vi "MAIN.vi"() -> ()   [LabVIEW 2020]
uses:
  GLOBALS.vi
panel:
  in  "Period 3":i64=20
  in  "Tab Control":enum32{"Page 1", "Page 2"}(tab)
  in  "reset":bool
  in  "Tecnica":bool
  out "PLOT_ALL":dynamicdata(graph)
  out "chaveamento":dbl
  out "HISTERESE":dbl(graph)
  out "termico":dbl
  out "TERMICO":dbl(graph)
  out "kalman_fused":dbl
  out "KALMAN_FUSED":dbl(graph)
  out "pitot":dbl
  out "Pitot? 2":bool
  out "Térmico?":bool
  out "Pitot?":bool
  out "PITOT":dbl(graph)
  in  "TERMICO Noise Amplitude":dbl=0.8
  in  "PITOT Noise Amplitude":dbl=2.0
  in  "Input":dbl(slide)=8.0 min=0.0 max=100.0 step=0.1 scale=0.0..100.0
  out "error":errorcluster
  in  "M":i32=10 min=2 max=100
  out "Térmico?":bool
  in  "hmin":dbl=8.0 min=5.0 max=20.0 step=1.0
  in  "hmax":dbl=11.0 min=6.0 max=14.0 step=1.0
  in  "stop":bool
  in  "gain delay termico\n[0,100]":dbl=93.0 min=0.0 max=100.0 step=1.0
  in  "Limpar_Graficos":bool
  in  "gain delay pitot [0,100]":dbl=50.0 min=0.0 max=100.0 step=1.0
  in  "PRINT":bool
  out "Kalman?":bool=TRUE
  in  "Ts [ms]":u32=200
  in  "saturacao_termico":dbl=15.0 format="%#_13g"
  # "Medidas Puras"
  # "Medidas Fundidas"
  # "Configurações\nda simulação"
  # "Chaveamento\ncom Histerese"
  # "Filtro de \nKalman"
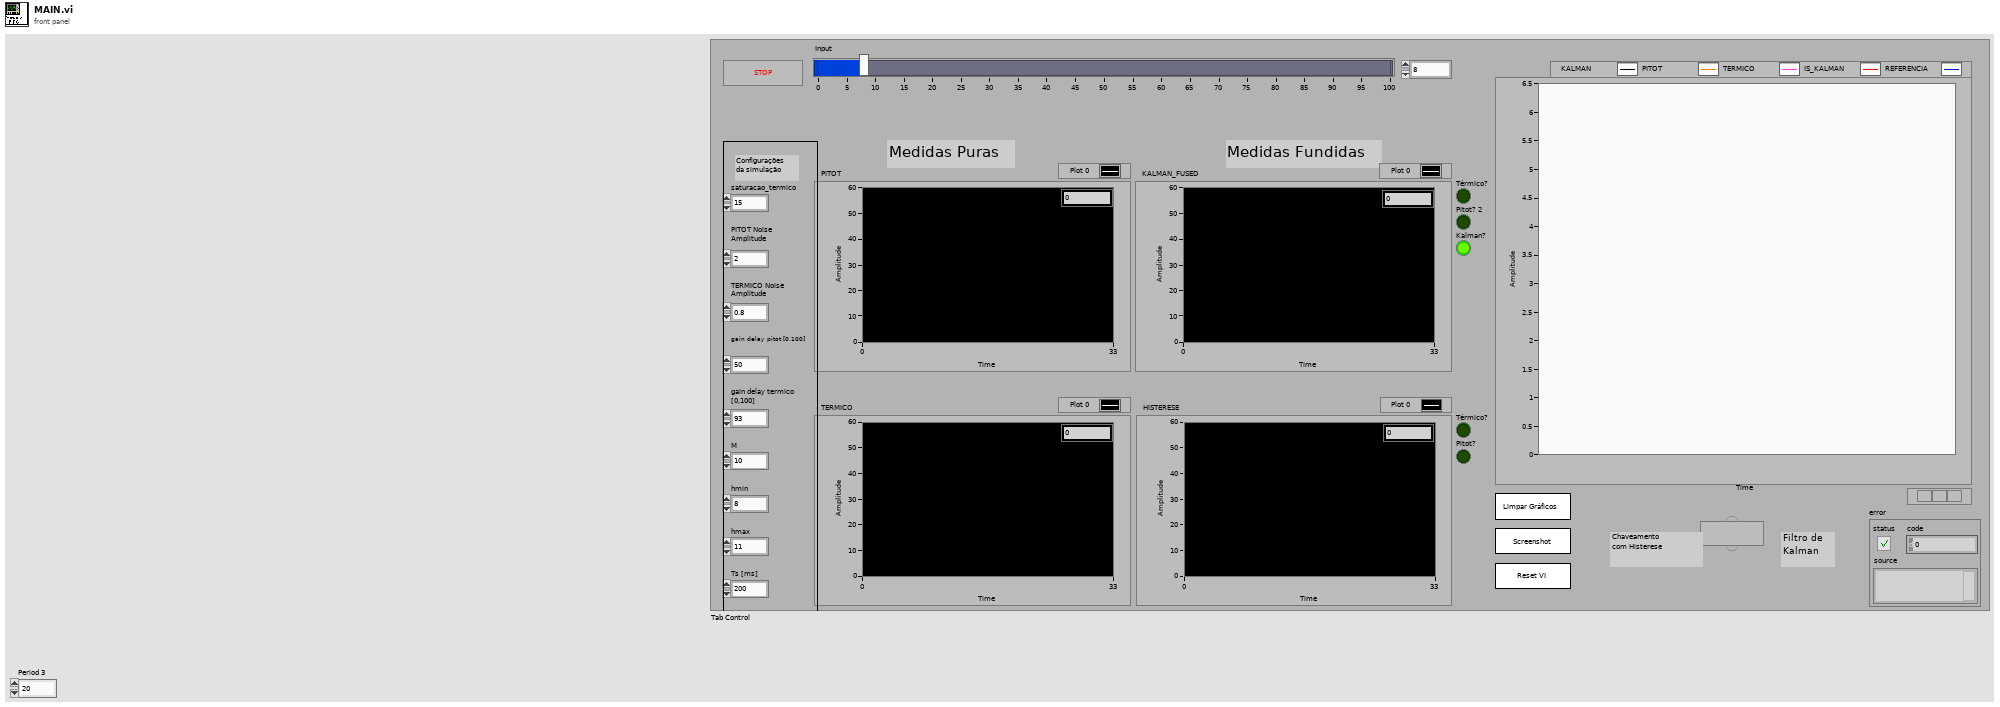
[diagram p1: front panel]
types:
  T1 = typedef "imagedata.ctl" = cluster{"image type":i32, "image depth":i32, "image":u8[], "mask":u8[], "colors":u32[], "Rectangle":cluster{"left":i16, "top":i16, "right":i16, "bottom":i16}}
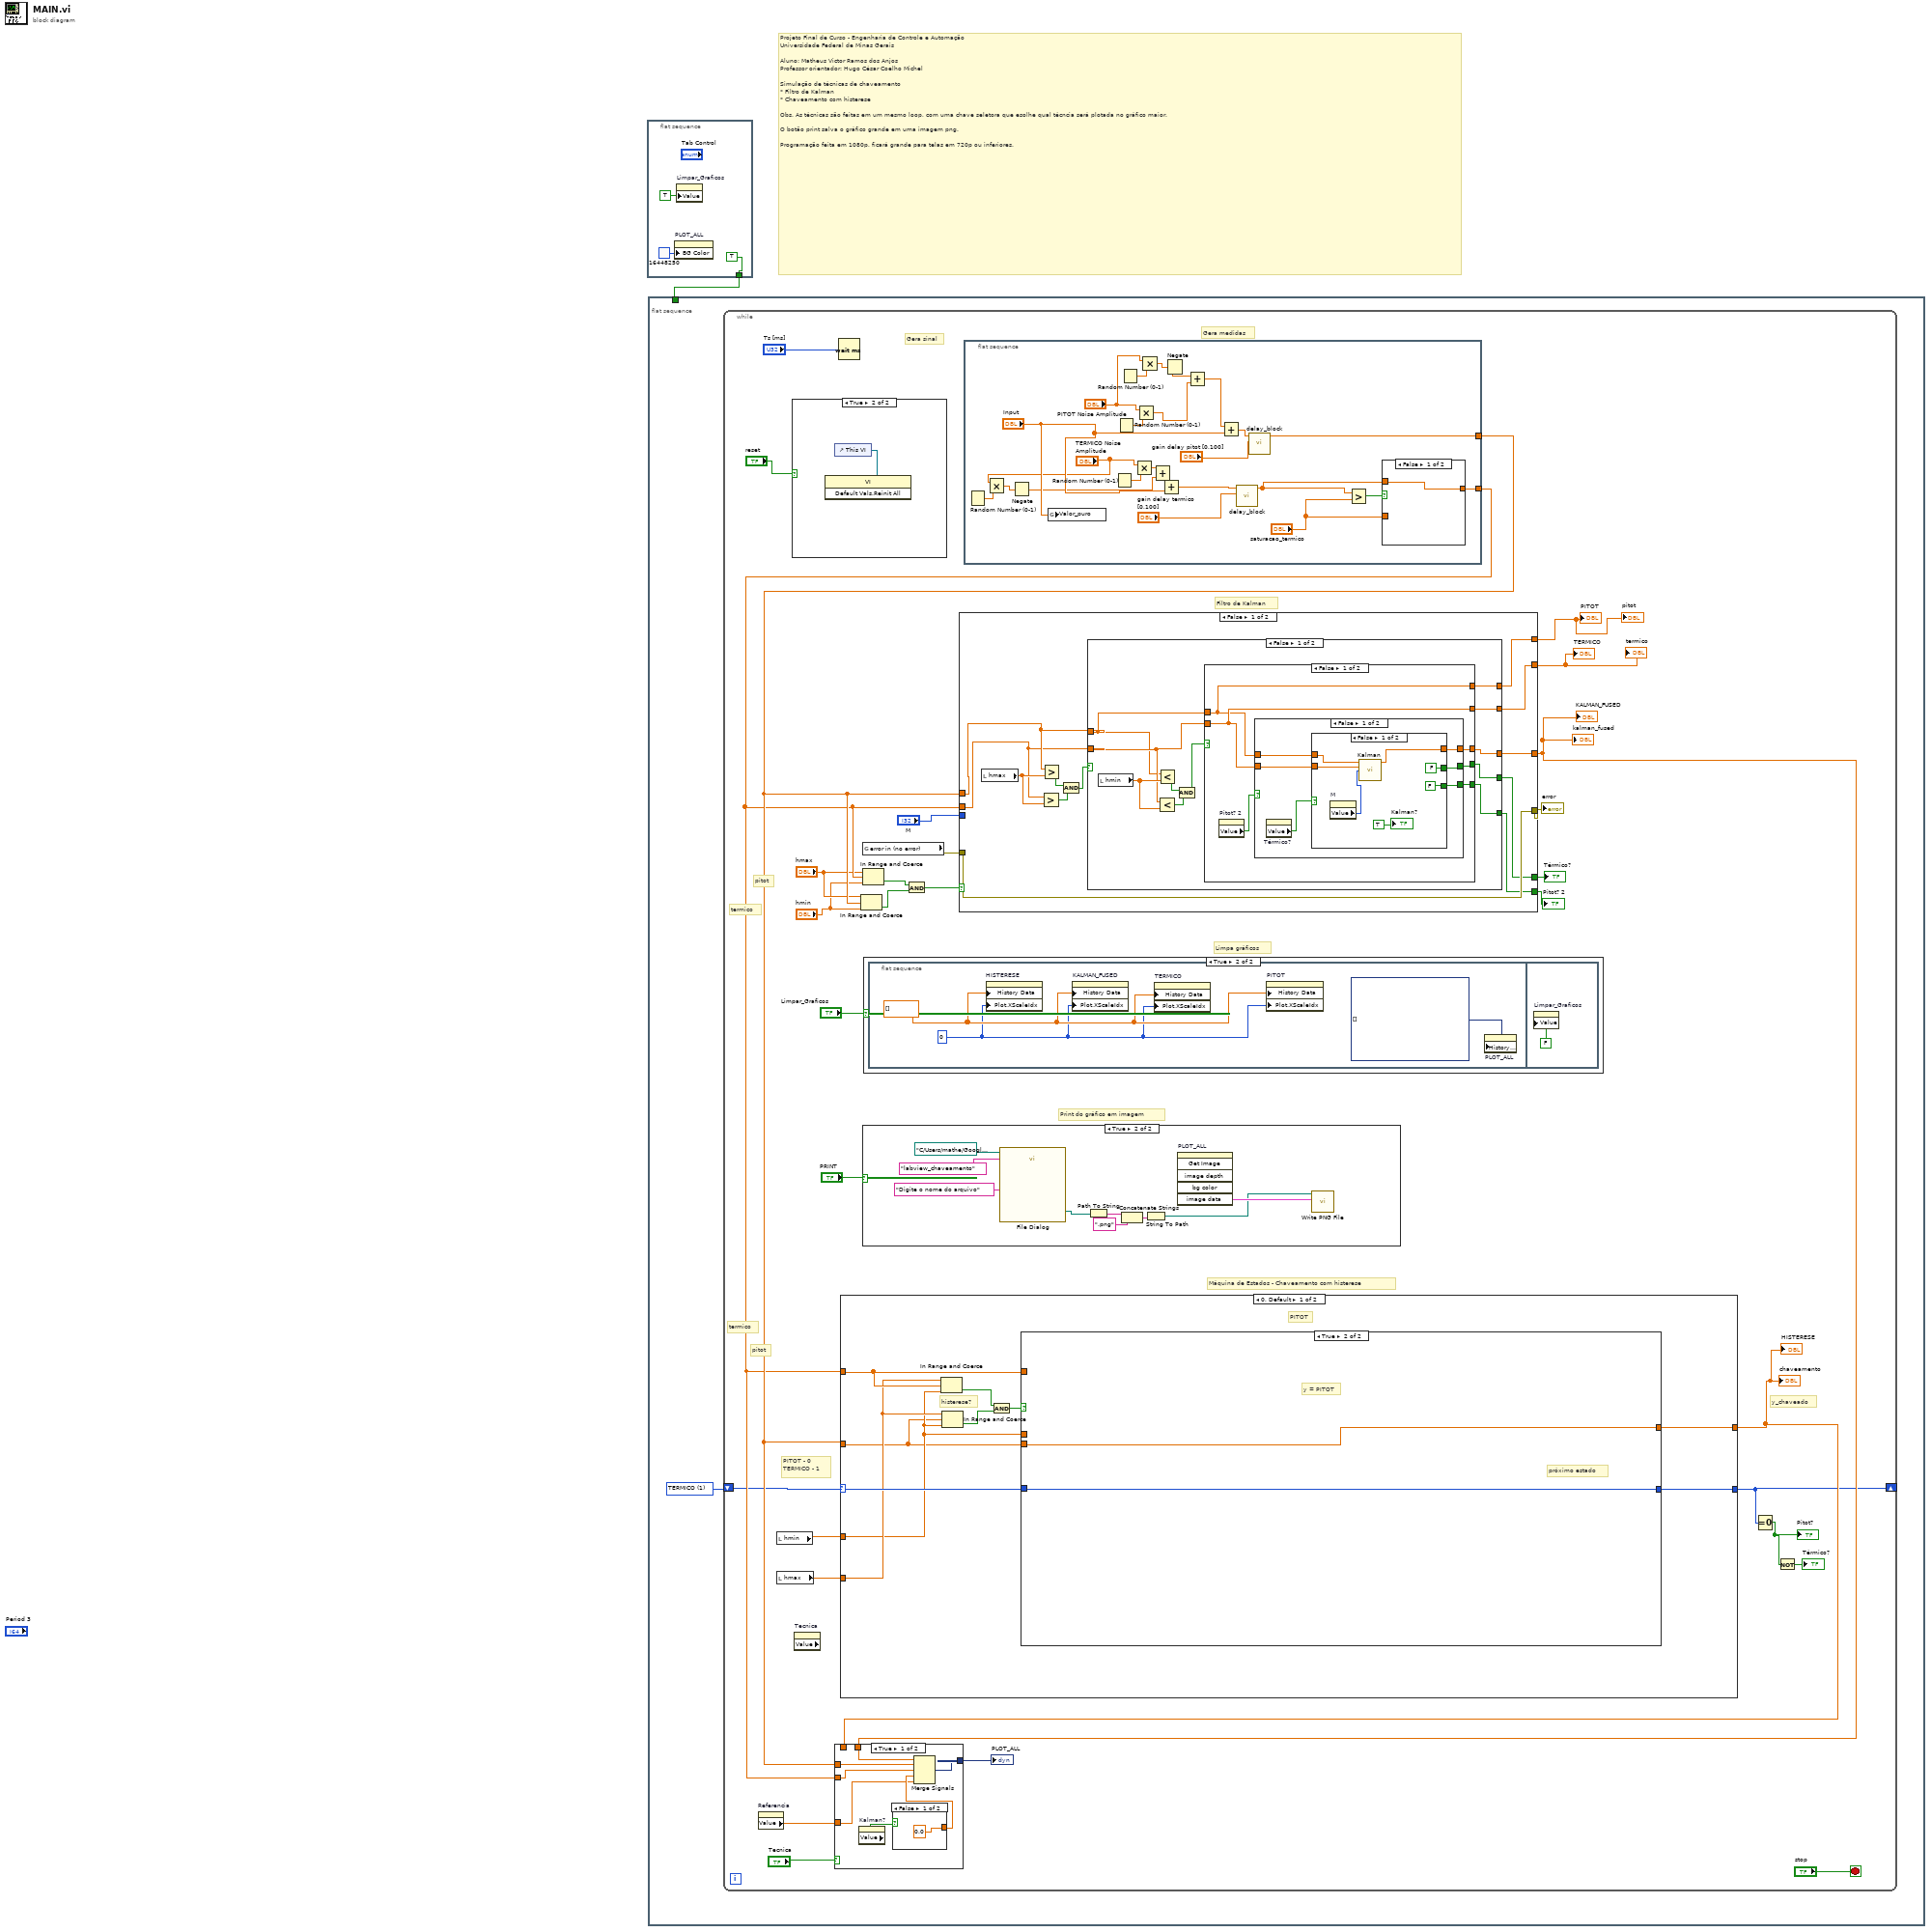
[diagram p0: block diagram]
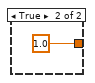
[diagram p4: hidden frame]
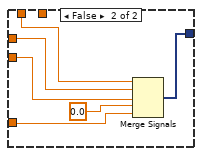
[diagram p5: hidden frame]
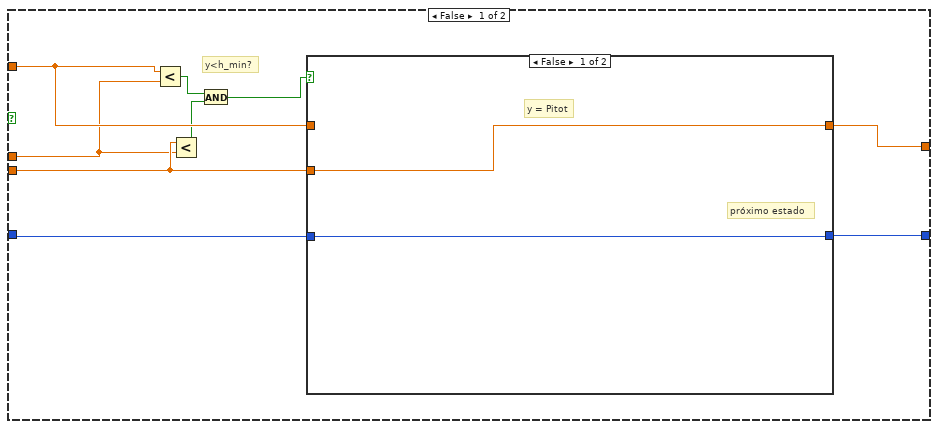
[diagram p6: hidden frame]
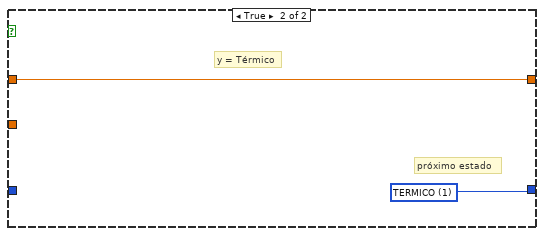
[diagram p7: hidden frame]
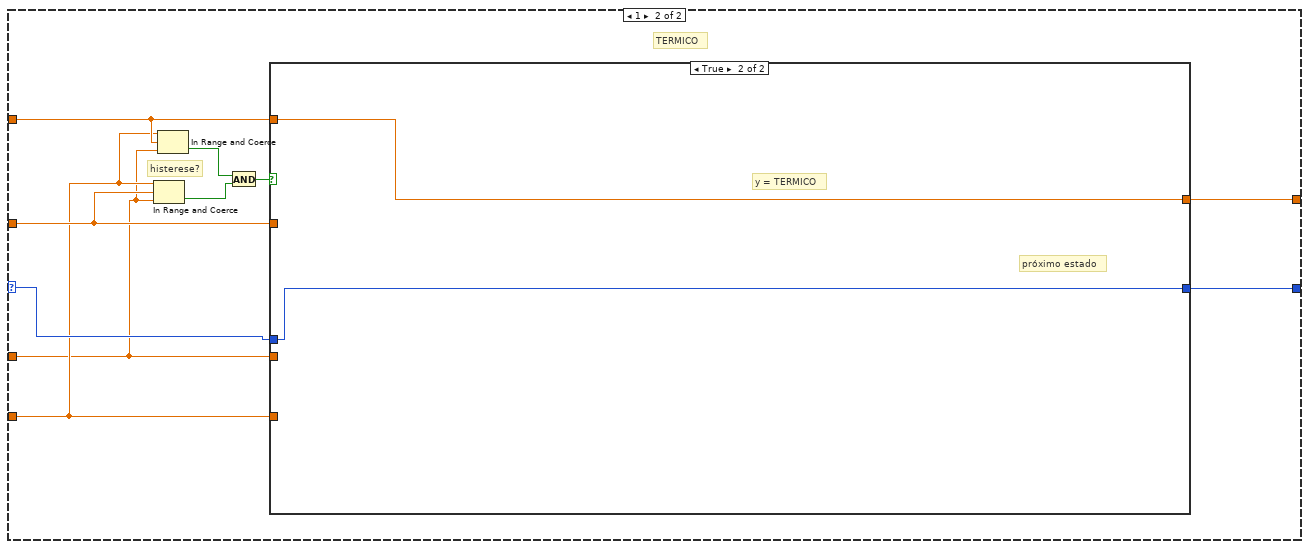
[diagram p8: hidden frame]
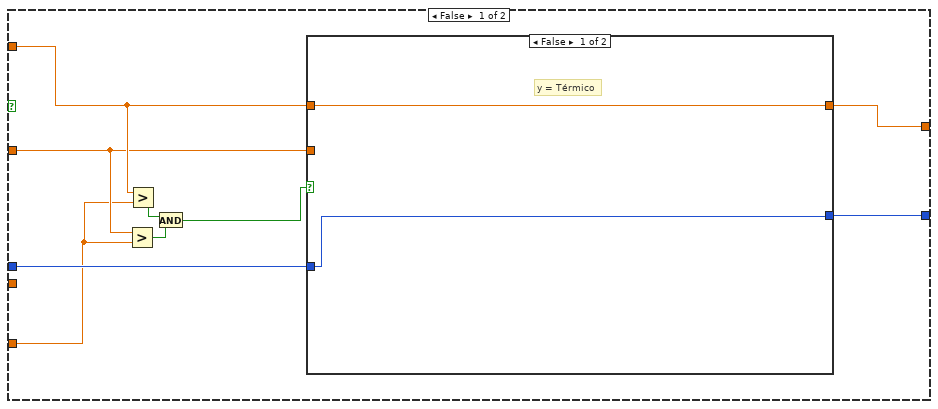
[diagram p9: hidden frame]
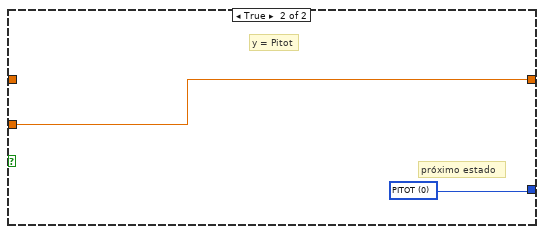
[diagram p10: hidden frame]
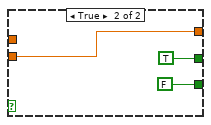
[diagram p13: hidden frame]
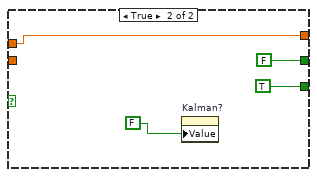
[diagram p14: hidden frame]
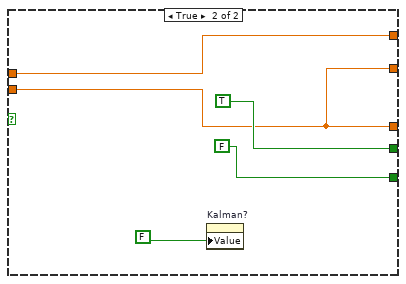
[diagram p15: hidden frame]
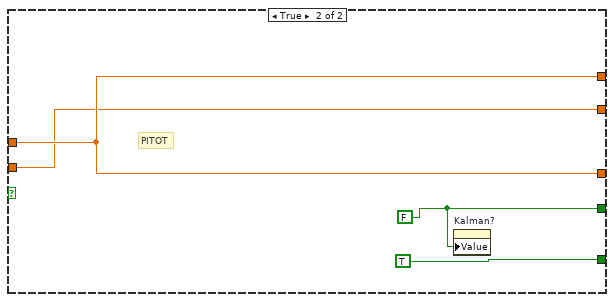
[diagram p16: hidden frame]
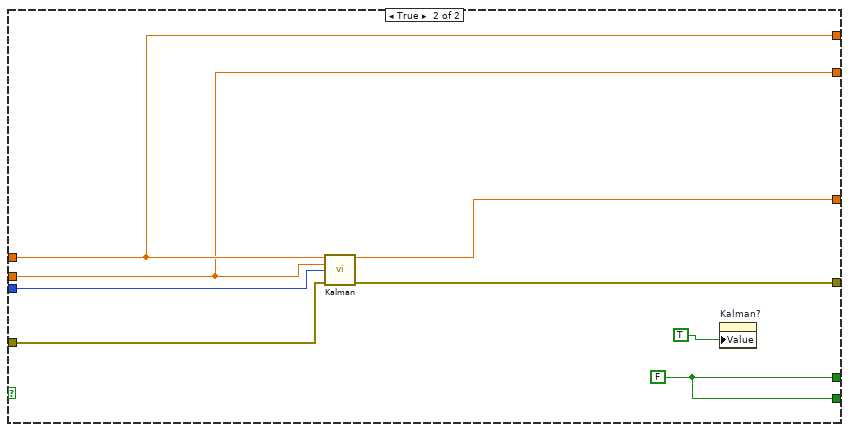
[diagram p17: hidden frame]
diagram:
  # "Projeto Final de Curso - Engenharia de Controle e Automação\nUniversidade Federal de Minas Gerais\n\nAluno: Matheus Victor Ramos dos Anjos\nProfessor orientador: Hugo César Coelho Michel\n\nSimulação de técnicas de chaveamento\n* Filtro de Kalman\n* Chaveamento com histerese\n\nObs. As técnicas são feitas em um mesmo loop, com uma chave seletora que esolhe qual técncia será plotada no gráfico maior.\n\nO botão print salva o gráfico grande em uma imagem png.\n\nProgramação feita em 1080p, ficará grande para telas em 720p ou inferiores."
  n1 = flat-sequence {
    tunnel: [TRUE] -> w1
    frame #0 {
      n2 = property on="PLOT_ALL" class="WFChart (strict)"("BG Color"=u32 16448250 ("Plot Area:Colors:BG Color")) -> ()  [unwired: 2 in, 2 out]
      n3 = property on="Limpar_Graficos" class="Bool (strict)"("Value"=TRUE ("Limpar_Graficos")) -> ()  [unwired: 2 in, 2 out]
    }
  }
  n4 = flat-sequence {
    tunnel: w1 -> [_]
    frame #0 {
      w5 = u16 1 items=["PITOT", "TERMICO"] ("Sensor_inicial")
      n5 = while {
        shift-right: [w7] -> _
        shift-left: w5 -> [w6]
        stop <- "stop" stop-if-true
        # "Gera medidas"
        # "Print do gráfico em imagem"
        # "Limpa gráficos"
        # "Máquina de Estados - Chaveamento com histerese"
        # "y_chaveado"
        # "Filtro de Kalman"
        # "Gera sinal"
        # "termico"
        # "pitot"
        # "pitot"
        # "termico"
        # "PITOT - 0\nTERMICO - 1"
        n6 = property on="Referencia" class="Slide (strict)"() -> ("Value"=w13:dbl)  [unwired: 2 in, 2 out]
        n7 = local read "hmin"() -> (w16:dbl)
        n8 = local read "hmax"() -> (w17:dbl)
        n9 = case shown="True" "reset" {
          frame False {
          }
          frame True {
            n10 = control-ref of="This VI"() -> (w62:refnum<vi>)
            n11 = invoke class="VI" method="Default Vals.Reinit All"(reference=w62) -> ()  [unwired: 2 in, 3 out]
          }
        }
        n12 = property on="Tecnica" class="Bool (strict)" props=["Value"]() -> ()  [unwired: 2 in, 3 out]
        n13 = Wait (ms)(milliseconds to wait="Ts [ms]") -> ()  [unwired: 1 out]
        n14 = case shown="0, Default" w6 {
          selector: w6 -> [w84 w109]
          tunnel: w16 -> [w82 w106]
          tunnel: w17 -> [w83 w107]
          tunnel: w34 -> [w86 w108]
          tunnel: w35 -> [w81 w110]
          tunnel: [w87 w112] -> w7
          tunnel: [w85 w111] -> w32
          frame 0, Default {
            # "histerese?"
            # "PITOT"
            n15 = In Range and Coerce(upper limit=w83, x=w86, lower limit=w82) -> (In Range?=w79:bool)  [unwired: 1 out]
            n16 = In Range and Coerce(upper limit=w83, x=w81, lower limit=w82) -> (In Range?=w80:bool)  [unwired: 1 out]
            n17 = And(x=w79, y=w80) -> (x .and. y?=w78:bool)
            n18 = case shown="True" w78 {
              tunnel: [w94 w102] -> w87
              tunnel: w86 -> [w96 _]
              tunnel: w81 -> [w92 w101]
              tunnel: [w95 w101] -> w85
              tunnel: w82 -> [w91 _]
              tunnel: w84 -> [w88 w102]
              frame False {
                # "y<h_min?"
                n19 = Less?(x=w96, y=w91) -> (x < y?=w93:bool)
                n20 = Less?(x=w92, y=w91) -> (x < y?=w90:bool)
                n21 = And(x=w93, y=w90) -> (x .and. y?=w89:bool)
                n22 = case shown="False" w89 {
                  tunnel: w96 -> [_ w100]
                  tunnel: w92 -> [w98 _]
                  tunnel: [w98 w100] -> w95
                  tunnel: [w97 w99] -> w94
                  tunnel: w88 -> [w97 _]
                  frame False {
                    # "próximo estado"
                    # "y = Pitot"
                  }
                  frame True {
                    w99 = u16 1 items=["PITOT", "TERMICO"] ("Sensor_inicial")
                    # "próximo estado"
                    # "y = Térmico"
                  }
                }
              }
              frame True {
                # "próximo estado"
                # "y = PITOT"
              }
            }
          }
          frame 1 {
            # "histerese?"
            # "TERMICO"
            n23 = In Range and Coerce(upper limit=w107, x=w110, lower limit=w106) -> (In Range?=w104:bool)  [unwired: 1 out]
            n24 = In Range and Coerce(upper limit=w107, x=w108, lower limit=w106) -> (In Range?=w105:bool)  [unwired: 1 out]
            n25 = And(x=w105, y=w104) -> (x .and. y?=w103:bool)
            n26 = case shown="True" w103 {
              tunnel: [w120 w127] -> w112
              tunnel: w108 -> [w117 w126]
              tunnel: w110 -> [w116 _]
              tunnel: [w121 w126] -> w111
              tunnel: w109 -> [w114 w127]
              tunnel: w107 -> [w113 _]
              tunnel: w106 -> [_ _]
              frame False {
                n27 = Greater?(x=w116, y=w113) -> (0:w118:bool)
                n28 = Greater?(x=w117, y=w113) -> (0:w119:bool)
                n29 = And(x=w119, y=w118) -> (x .and. y?=w115:bool)
                n30 = case shown="False" w115 {
                  tunnel: w117 -> [w123 _]
                  tunnel: w116 -> [_ w125]
                  tunnel: [w123 w125] -> w121
                  tunnel: [w122 w124] -> w120
                  tunnel: w114 -> [w122 _]
                  frame False {
                    # "y = Térmico"
                  }
                  frame True {
                    w124 = u16 0 items=["PITOT", "TERMICO"] ("Sensor_inicial")
                    # "próximo estado"
                    # "y = Pitot"
                  }
                }
              }
              frame True {
                # "próximo estado"
                # "y = TERMICO"
              }
            }
          }
        }
        "chaveamento" <- w32
        "HISTERESE" <- w32
        n31 = In Range and Coerce(upper limit="hmax", x=w35, lower limit="hmin") -> (In Range?=w19:bool)  [unwired: 1 out]
        n32 = global read "GLOBALS.vi" "error in (no error)"() -> (w31:errorcluster)
        n33 = In Range and Coerce(upper limit="hmax", x=w34, lower limit="hmin") -> (In Range?=w18:bool)  [unwired: 1 out]
        n34 = case shown="True" "PRINT" {
          frame False {
          }
          frame True {
            n35 = call "File Dialog"("start path"=path "C:/Users/mathe/Google Drive/PFC - Matheus Ramos/Monografia/Imagens/labview", "prompt"="Digite o nome do arquivo", "default name"="labview_chaveamento") -> ("selected path"=w133:path)  [unwired: 9 in, 3 out]
            n36 = Path To String(path=w133) -> (string=w132:string)
            n37 = Concatenate Strings(w132, ".png" ("string")) -> (w130:string)
            n38 = String To Path(string=w130) -> (path=w128:path)
            n39 = invoke on="PLOT_ALL" class="WFChart (strict)" method="Get Image"() -> ("image data"=w129:T1)  [unwired: 6 in, 5 out]
            n40 = call <vilib>:"Write PNG File.vi"("image data"=w129, "path to PNG file"=w128) -> ()  [unwired: 8 in, 2 out]
          }
        }
        n41 = case shown="True" "Limpar_Graficos" {
          frame False {
          }
          frame True {
            n42 = flat-sequence {
              frame #0 {
                w138 = u32 0 ("Plot.X Scale Index")
                w139 = dbl[] [] ("History Data")
                n43 = property on="HISTERESE" class="WFChart (strict)"("History Data"=w139, "Plot.XScaleIdx"=w138) -> ()  [unwired: 2 in, 2 out]
                n44 = property on="KALMAN_FUSED" class="WFChart (strict)"("History Data"=w139, "Plot.XScaleIdx"=w138) -> ()  [unwired: 2 in, 2 out]
                n45 = property on="TERMICO" class="WFChart (strict)"("History Data"=w139, "Plot.XScaleIdx"=w138) -> ()  [unwired: 2 in, 2 out]
                n46 = property on="PITOT" class="WFChart (strict)"("History Data"=w139, "Plot.XScaleIdx"=w138) -> ()  [unwired: 2 in, 2 out]
                n47 = property on="PLOT_ALL" class="WFChart (strict)"("History Data"=dynamicdata[] []) -> ()  [unwired: 2 in, 2 out]
              }
              frame #1 {
                n48 = property on="Limpar_Graficos" class="Bool (strict)"("Value"=FALSE ("Limpar_Graficos")) -> ()  [unwired: 2 in, 2 out]
              }
            }
          }
        }
        n49 = And(x=w18, y=w19) -> (x .and. y?=w28:bool)
        n50 = case shown="False" w28 {
          tunnel: w31 -> [w152 w206]
          tunnel: "M" -> [_ w205]
          tunnel: [w152 w204] -> w29
          tunnel: [w145 w203] -> w33
          tunnel: w35 -> [w142 w200]
          tunnel: w34 -> [w141 w199]
          tunnel: [w147 w202] -> w27
          tunnel: [w148 w202] -> w26
          tunnel: [w144 w200] -> w23
          tunnel: [w143 w199] -> w22
          frame False {
            n51 = local read "hmax"() -> (w146:dbl)
            n52 = Greater?(x=w141, y=w146) -> (0:w150:bool)
            n53 = Greater?(x=w142, y=w146) -> (0:w151:bool)
            n54 = And(x=w151, y=w150) -> (x .and. y?=w149:bool)
            n55 = case shown="False" w149 {
              tunnel: [w158 w197] -> w148
              tunnel: [w159 TRUE] -> w147
              tunnel: [w156 w196] -> w145
              tunnel: w142 -> [w155 w196]
              tunnel: w141 -> [w157 w195]
              tunnel: [w154 w196] -> w144
              tunnel: [w153 w195] -> w143
              frame False {
                n56 = local read "hmin"() -> (w160:dbl)
                n57 = Less?(x=w157, y=w160) -> (x < y?=w163:bool)
                n58 = Less?(x=w155, y=w160) -> (x < y?=w162:bool)
                n59 = And(x=w162, y=w163) -> (x .and. y?=w161:bool)
                n60 = case shown="False" w161 {
                  tunnel: [w168 TRUE] -> w158
                  tunnel: [w167 FALSE] -> w159
                  tunnel: w157 -> [w165 w190]
                  tunnel: [w166 w190] -> w156
                  tunnel: w155 -> [w164 w191]
                  tunnel: [w164 w191] -> w154
                  tunnel: [w165 w190] -> w153
                  frame False {
                    n61 = property on="Pitot? 2" class="Bool (strict)"() -> ("Value"=w169:bool)  [unwired: 2 in, 2 out]
                    n62 = case shown="False" w169 {
                      tunnel: w165 -> [w174 _]
                      tunnel: w164 -> [w173 w187]
                      tunnel: [w172 FALSE] -> w168
                      tunnel: [w171 TRUE] -> w167
                      tunnel: [w170 w187] -> w166
                      frame False {
                        n63 = property on="Térmico?" class="Bool (strict)"() -> ("Value"=w175:bool)  [unwired: 2 in, 2 out]
                        n64 = case shown="False" w175 {
                          tunnel: w174 -> [w178 w183]
                          tunnel: w173 -> [w179 _]
                          tunnel: [FALSE TRUE] -> w172
                          tunnel: [FALSE FALSE] -> w171
                          tunnel: [w176 w183] -> w170
                          frame False {
                            n65 = property on="M" class="DigNum (strict)"() -> ("Value"=w177:i32)  [unwired: 2 in, 2 out]
                            n66 = call "Kalman.vi"("y1"=w179, "y2"=w178, "M"=w177) -> ("y_fused"=w176:dbl)  [unwired: 7 in, 5 out]
                            "Kalman?" <- TRUE
                          }
                          frame True {
                          }
                        }
                      }
                      frame True {
                        n67 = property on="Kalman?" class="Bool (strict)"("Value"=FALSE) -> ()  [unwired: 2 in, 2 out]
                      }
                    }
                  }
                  frame True {
                    n68 = property on="Kalman?" class="Bool (strict)"("Value"=FALSE ("Kalman?")) -> ()  [unwired: 2 in, 2 out]
                  }
                }
              }
              frame True {
                w197 = FALSE
                # "PITOT"
                n69 = property on="Kalman?" class="Bool (strict)"("Value"=w197) -> ()  [unwired: 2 in, 2 out]
              }
            }
          }
          frame True {
            w202 = FALSE
            n70 = call "Kalman.vi"("y1"=w200, "y2"=w199, "M"=w205, "error in (no error)"=w206) -> ("y_fused"=w203:dbl, "error out"=w204:errorcluster)  [unwired: 6 in, 4 out]
            n71 = property on="Kalman?" class="Bool (strict)"("Value"=TRUE) -> ()  [unwired: 2 in, 2 out]
          }
        }
        "error" <- w29
        "Térmico?" <- w26
        "Pitot? 2" <- w27
        "kalman_fused" <- w33
        "KALMAN_FUSED" <- w33
        "PITOT" <- w23
        "pitot" <- w23
        "termico" <- w22
        "TERMICO" <- w22
        n72 = case shown="True" "Tecnica" {
          tunnel: w33 -> [w69 _]
          tunnel: [w68 w77] -> w11
          tunnel: w35 -> [w65 w74]
          tunnel: w34 -> [w64 w73]
          tunnel: w13 -> [w63 w75]
          tunnel: w32 -> [_ w72]
          frame True {
            n73 = property on="Kalman?" class="Bool (strict)"() -> ("Value"=w66:bool)  [unwired: 2 in, 2 out]
            n74 = case shown="False" w66 {
              tunnel: [0.0 1.0] -> w67
              frame False {
              }
              frame True {
              }
            }
            n75 = Merge Signals(w69, w65, w64, w67, w63) -> (w68:dynamicdata)
          }
          frame False {
            n76 = Merge Signals(w72, w74, w73, 0.0, w75) -> (w77:dynamicdata)
          }
        }
        "PLOT_ALL" <- w11
        n77 = flat-sequence {
          tunnel: [w59] -> w35
          tunnel: [w58] -> w34
          frame #0 {
            n78 = Random Number (0-1)() -> (number: 0 to 1=w41:dbl)
            n79 = Multiply(x="TERMICO Noise Amplitude", y=w41) -> (x*y=w40:dbl)
            n80 = Negate(x=w40) -> (-x=w36:dbl)
            n81 = global write "GLOBALS.vi" "Valor_puro"("Input") -> ()
            n82 = Random Number (0-1)() -> (number: 0 to 1=w56:dbl)
            n83 = Random Number (0-1)() -> (number: 0 to 1=w57:dbl)
            n84 = Random Number (0-1)() -> (number: 0 to 1=w47:dbl)
            n85 = Multiply(x="TERMICO Noise Amplitude", y=w56) -> (x*y=w38:dbl)
            n86 = Multiply(x="PITOT Noise Amplitude", y=w57) -> (x*y=w44:dbl)
            n87 = Multiply(x="PITOT Noise Amplitude", y=w47) -> (x*y=w46:dbl)
            n88 = Add(x=w38, y=w36) -> (x+y=w37:dbl)
            n89 = Add(x=w37, y="Input") -> (x+y=w54:dbl)
            n90 = Negate(x=w46) -> (-x=w45:dbl)
            n91 = Add(x=w45, y=w44) -> (x+y=w43:dbl)
            n92 = Add(x=w43, y="Input") -> (x+y=w52:dbl)
            n93 = call "delay_block.vi"("gain"="gain delay termico\n[0,100]", "signal"=w54) -> ("signal_out"=w49:dbl)  [unwired: 9 in]
            n94 = call "delay_block.vi"("gain"="gain delay pitot [0,100]", "signal"=w52) -> ("signal_out"=w59:dbl)  [unwired: 9 in]
            n95 = Greater?(x=w49, y="saturacao_termico") -> (0:w55:bool)
            n96 = case shown="False" w55 {
              tunnel: "saturacao_termico" -> [_ w61]
              tunnel: [w60 w61] -> w58
              tunnel: w49 -> [w60 _]
              frame False {
              }
              frame True {
              }
            }
          }
        }
        n97 = Equal To 0?(x=w7) -> (x = 0?=w14:bool)
        "Pitot?" <- w14
        n98 = Not(x=w14) -> (.not. x?=→"Térmico?":bool)
      }
    }
  }
